vi "Current_Calib_Filenames.vi"(3 "Calib Filename":path[](array[path]), 4 "Channel Numbers":i16[](array[numeric]) min=0 max=7, 5 "Mode":T1) -> (0 "Calib Filename Out":path[](array[path]), 1 "Channel Numbers Out":i16[](array[numeric]) min=0 max=7)   [LabVIEW 2010]
uses:
  Controls/App_Global.ctl
  File/Setup_Filetype.ctl
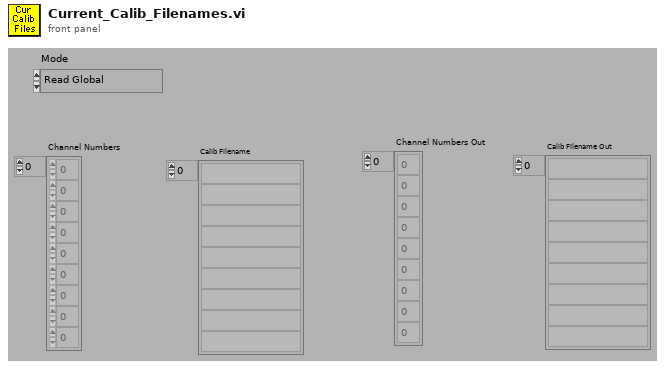
[diagram p1: front panel]
types:
  T1 = typedef "App_Global.ctl" = enum16{"Read Global", "Write to Global", "Initialise Array"}
  T2 = typedef "Setup_Filetype.ctl" = enum16{"Measurement Setups", "Calibration Setups", "General", "Results File Plotter Setups", "Speed Calib Tweaks"}
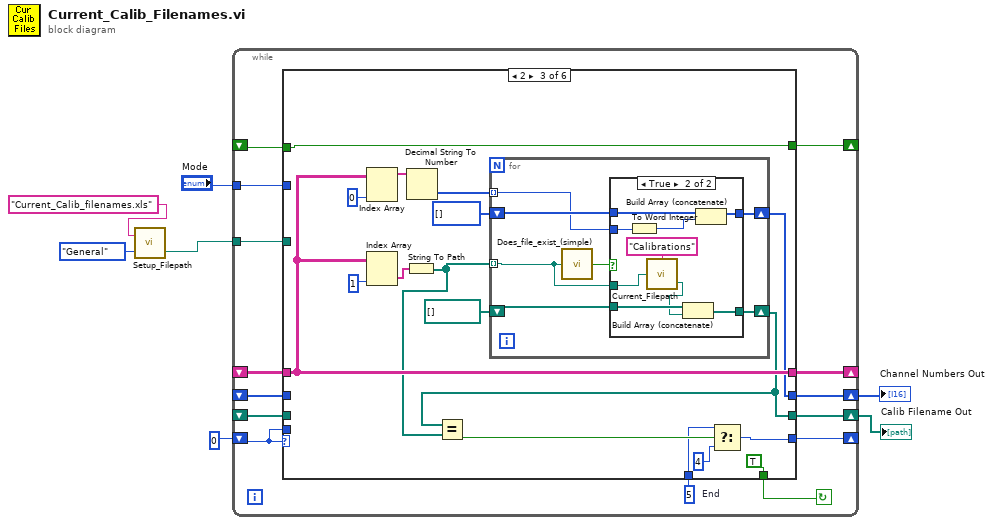
[diagram p0: block diagram]
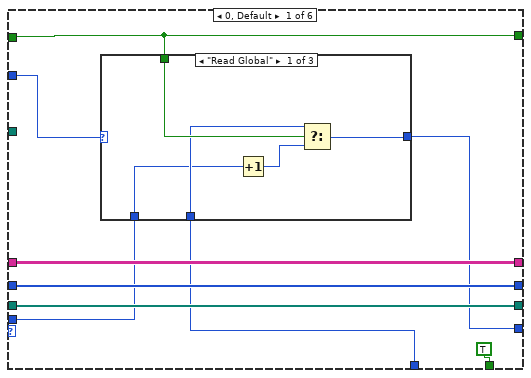
[diagram p2: hidden frame]
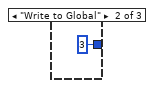
[diagram p3: hidden frame]
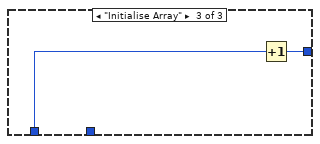
[diagram p4: hidden frame]
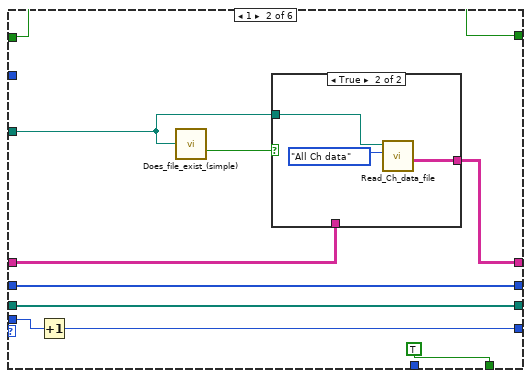
[diagram p5: hidden frame]
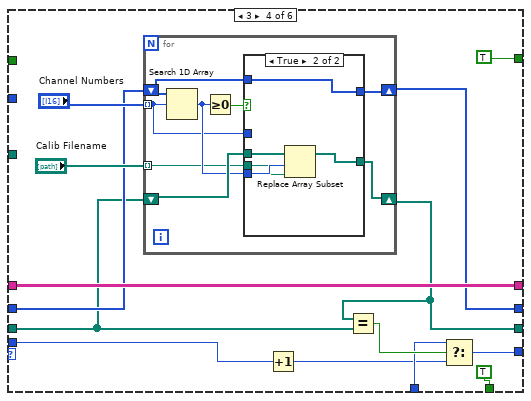
[diagram p8: hidden frame]
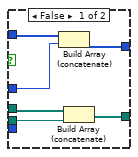
[diagram p9: hidden frame]
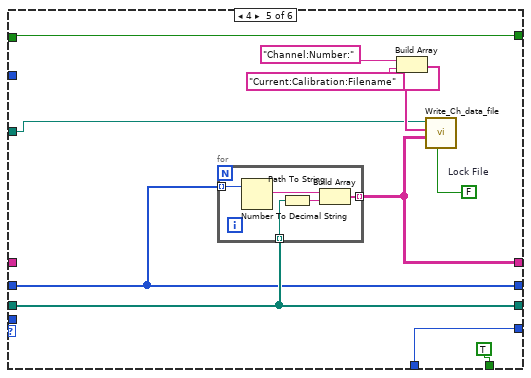
[diagram p10: hidden frame]
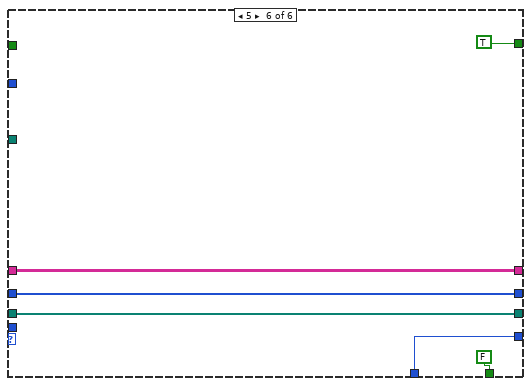
[diagram p11: hidden frame]
diagram:
  n1 = call "Setup_Filepath.vi"("Setup File Type"=Setup_Filetype."General", "Filename in"="Current_Calib_filenames.xls" ("Substring")) -> ("Filename Out"=w2:path)  [unwired: 1 out]
  n2 = while {
    shift-left: _ -> [w10]
    shift-right: [w12] -> w4
    shift-left: _ -> [w11]
    shift-right: [w13] -> w5
    tunnel: "Mode" -> [w17]
    shift-left: 0 -> [w18]
    shift-right: [w19] -> _
    shift-left: _ -> [w14]
    shift-right: [w15] -> _
    shift-left: _ -> [w21]
    shift-right: [w16] -> _
    tunnel: w2 -> [w8]
    stop <- w20 continue-if-true
    w9 = 5  # End
    n3 = case shown="2" w18 {
      tunnel: w21 -> [w25 w45 w64 _ w131 _]
      tunnel: [TRUE TRUE TRUE TRUE TRUE FALSE] -> w20
      tunnel: [w22 w46 w55 w88 w130 w138] -> w19
      tunnel: w18 -> [w23 w47 _ w90 _ _]
      tunnel: w17 -> [w26 _ _ _ _ _]
      tunnel: [w25 w45 w64 TRUE w131 TRUE] -> w16
      tunnel: [w28 w43 w63 w100 w123 w141] -> w15
      tunnel: w14 -> [w28 w42 w63 w100 _ w141]
      tunnel: [w30 w41 w60 w95 w124 w140] -> w13
      tunnel: [w29 w40 w59 w94 w125 w139] -> w12
      tunnel: w11 -> [w30 w41 _ w96 w124 w140]
      tunnel: w10 -> [w29 w40 _ w93 w125 w139]
      tunnel: w9 -> [w24 _ w56 w91 w130 w138]
      tunnel: w8 -> [_ w39 _ _ w121 _]
      frame 0, Default {
        n4 = case shown="\"Read Global\"" w26 {
          tunnel: w25 -> [w35 _ _]
          tunnel: w24 -> [w34 _ _]
          tunnel: w23 -> [w32 _ w38]
          tunnel: [w31 3 ("End") w37] -> w22
          frame "Read Global" {
            n5 = Increment(x=w32) -> (x+1=w33:i32)
            n6 = Select(t=w34, s=w35, f=w33) -> (s? t:f=w31:i32)
          }
          frame "Write to Global" {
          }
          frame "Initialise Array" {
            n7 = Increment(x=w38) -> (x+1=w37:i32)
          }
        }
      }
      frame 1 {
        n8 = Increment(x=w47) -> (x+1=w46:i32)
        n9 = call "Does_file_exist_(simple).vi"("Pathname"=w39) -> ("exists?"=w44:bool)
        n10 = case shown="True" w44 {
          tunnel: w39 -> [_ w51]
          tunnel: [w49 w50] -> w43
          tunnel: w42 -> [w49 _]
          frame False {
          }
          frame True {
            n11 = call "Read_Ch_data_file.vi"("Output"=enum16{"All Ch data", "The last few rows"}."All Ch data", "Filename"=w51) -> ("Channel Values"=w50:string[][])  [unwired: 3 in, 4 out]
          }
        }
      }
      frame 2 {
        n12 = Index Array(array=w63, index (col)=0 ("Index")) -> (element=w66:string[])  [unwired: 1 in]
        n13 = Index Array(array=w63, index (col)=1 ("Index")) -> (element=w65:string[])  [unwired: 1 in]
        n14 = String To Path(string=w65) -> (path=w58:path[])
        n15 = Decimal String To Number(string=w66) -> (number=w53:i32[])  [unwired: 3 out]
        n16 = for {
          shift-right: [w74] -> w60
          shift-right: [w71] -> w59
          shift-left: path[] [] -> [w72]
          tunnel: w58 -> [w70] mode=indexing
          shift-left: i16[] [] -> [w75]
          tunnel: w53 -> [w73] mode=indexing
          n17 = call "Does_file_exist_(simple).vi"("Pathname"=w70) -> ("exists?"=w76:bool)
          n18 = case shown="True" w76 {
            tunnel: w75 -> [w78 w87]
            tunnel: [w78 w86] -> w74
            tunnel: w73 -> [_ w83]
            tunnel: w72 -> [w77 w85]
            tunnel: [w77 w84] -> w71
            tunnel: w70 -> [_ w81]
            frame False {
            }
            frame True {
              n19 = To Word Integer(number=w83) -> (16bit integer=w82:i16)
              n20 = call "Current_Filepath.vi"("Filename in"=w81, "Data Type"="Calibrations") -> ("Filename Out"=w79:path)  [unwired: 1 out]
              n21 = Build Array (concatenate)(w85, w79) -> (w84:path[])
              n22 = Build Array (concatenate)(w87, w82) -> (w86:i16[])
            }
          }
        }
        n23 = Equal?(x=w59, y=w58) -> (x = y?=w57:bool)
        n24 = Select(t=w56, s=w57, f=4) -> (s? t:f=w55:i32)
      }
      frame 3 {
        n25 = for {
          tunnel: "Channel Numbers" -> [w102] mode=indexing
          shift-right: [w105] -> w94
          shift-left: w93 -> [w108]
          tunnel: "Calib Filename" -> [w106] mode=indexing
          shift-right: [w104] -> w95
          shift-left: w96 -> [w103]
          n26 = Search 1D Array(1D array=w103, element=w102) -> (index of element=w107:i32)  [unwired: 1 out]
          n27 = Greater Or Equal To 0?(x=w107) -> (x >= 0?=w109:bool)
          n28 = case shown="True" w109 {
            tunnel: w108 -> [w112 w120]
            tunnel: w107 -> [_ w119]
            tunnel: w106 -> [w111 w118]
            tunnel: [w110 w117] -> w105
            tunnel: [w113 w116] -> w104
            tunnel: w103 -> [w115 w116]
            tunnel: w102 -> [w114 _]
            frame False {
              n29 = Build Array (concatenate)(w115, w114) -> (w113:i16[])
              n30 = Build Array (concatenate)(w112, w111) -> (w110:path[])
            }
            frame True {
              n31 = Replace Array Subset(array=w120, new element=w118, index=w119) -> (w117:path[])
            }
          }
        }
        n32 = Increment(x=w90) -> (x+1=w89:i32)
        n33 = Equal?(x=w94, y=w93) -> (x = y?=w92:bool)
        n34 = Select(t=w91, s=w92, f=w89) -> (s? t:f=w88:i32)
      }
      frame 4 {
        w122 = FALSE  # Lock File
        n35 = for {
          tunnel: w125 -> [w136] mode=indexing
          tunnel: w124 -> [w135] mode=indexing
          tunnel: [w133] -> w123 mode=indexing
          n36 = Number To Decimal String(number=w135) -> (decimal integer string=w134:string)  [unwired: 1 out]
          n37 = Path To String(path=w136) -> (string=w132:string)
          n38 = Build Array(w134, w132) -> (w133:string[])
        }
        n39 = Build Array("Channel:Number:", "Current:Calibration:Filename") -> (w126:string[])
        n40 = call "Write_Ch_data_file.vi"("Lock File"=w122, "Channel Values"=w123, "Channel names"=w126, "Filename"=w121) -> ()  [unwired: 4 in, 4 out]
      }
      frame 5 {
      }
    }
  }
  "Channel Numbers Out" <- w5
  "Calib Filename Out" <- w4
